vi "GetType.vi"(8 "error in (no error)":errorcluster, 11 "Set Ratios Msg":refnum<class "Set Ratios Msg.lvclass">) -> (0 "error out":errorcluster, 2 "Data Sample":variant, 3 "Set Ratios Msg":refnum<class "Set Ratios Msg.lvclass">)   [LabVIEW 2020, in "BNT_ULx.lvlib" / "Set Ratios Msg.lvclass"]
uses:
  Set Ratios Msg.lvclass
  Set Ratios Msg.lvclass/Set Ratios Msg.ctl
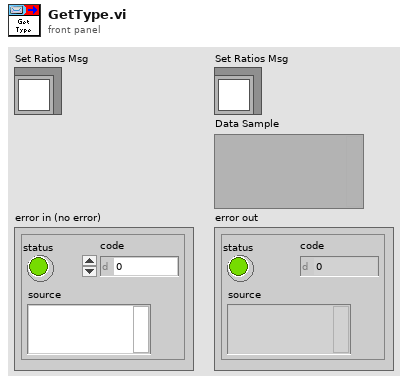
[diagram p1: front panel]
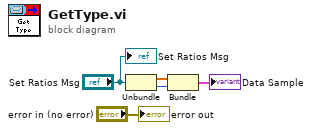
[diagram p0: block diagram]
diagram:
  n1 = Unbundle("Set Ratios Msg") -> (w2:dbl[], w1:i32)
  n2 = Bundle("PWM Ratios"=w2, "Start Index"=w1) -> (→"Data Sample":cluster{"PWM Ratios":dbl[], "Start Index":i32})  [unwired: 1 in]
  "error out" <- "error in (no error)"
  "Set Ratios Msg" <- "Set Ratios Msg"
